vi "Go To Connecting.vi"(8 "error in (no error)":errorcluster, 11 "ConnectCommand in":refnum<class "Connect Command.lvclass">=refnum) -> (0 "error out":errorcluster, 3 "State Actor.lvclass":refnum<class "State Actor.lvclass">)   [LabVIEW 2013, in "Receiver.lvlib" / "Receive Commands Using State Actors.lvlib" / "Connect Command.lvlib" / "Connect Command.lvclass"]
uses:
  Connect Command/Connect Command.lvclass
  <vilib>/ni/Actors/State Actor/State Actor/State Actor.lvclass
  ReceiverConnectingState/Connecting.lvclass
  <vilib>/ActorFramework/Actor/Actor.lvclass/Actor.ctl
  <vilib>/ActorFramework/Message Enqueuer/Message Enqueuer.lvclass/Message Enqueuer.ctl
  <vilib>/ActorFramework/Message Enqueuer/Init from Existing Queue.vi
  <vilib>/ActorFramework/Message Enqueuer/Enqueue.vi
  <vilib>/ActorFramework/Message Priority Queue/Priority Enqueue.vi
  <vilib>/ActorFramework/Message Enqueuer/Message Enqueuer.lvclass
  Command Messages/Start Command Msg/Start Command Msg.lvclass
  <vilib>/ActorFramework/Actor/Actor.lvclass
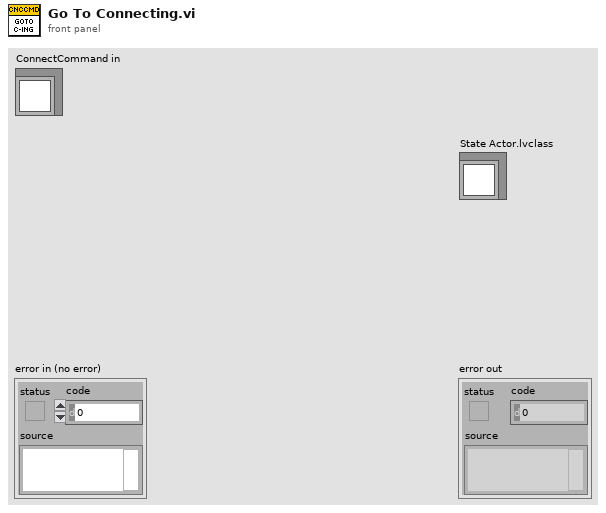
[diagram p1: front panel]
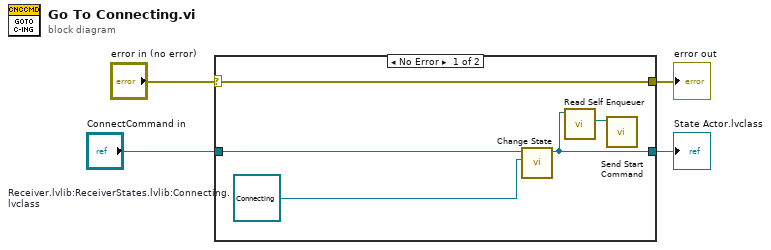
[diagram p0: block diagram]
diagram:
  n1 = case shown="No Error" "error in (no error)" {
    selector: "error in (no error)" -> [w9 w11]
    tunnel: [w9 w11] -> w3
    tunnel: [w6 w10] -> w1
    tunnel: "ConnectCommand in" -> [w7 w10]
    frame No Error {
      w8 = refnum<class "Connecting.lvclass"> refnum  # Receiver.lvlib:ReceiverStates.lvlib:Connecting.lvclass
      n2 = call <vilib>:"Change State.vi"("New State in"=w8, "State in"=w7) -> ("State out"=w6:refnum<class "State Actor.lvclass">)  [unwired: 8 in, 1 out]
      n3 = call <vilib>:"Read Self Enqueuer.vi"("Actor"=w6) -> ("Self Enqueuer"=w5:refnum<class "Message Enqueuer.lvclass">)  [unwired: 10 in]
      n4 = call "Send Start Command.vi"("Message Enqueuer"=w5) -> ()  [unwired: 9 in, 2 out]
    }
    frame Error {
    }
  }
  "error out" <- w3
  "State Actor.lvclass" <- w1
